vi "Run Test.vi"(8 "error in (no error)":errorcluster, 11 "Test Template in":refnum<class "LCM Single-Up APP Programming.lvclass">) -> (0 "error out":errorcluster, 1 "Fail Codes":string[](array[string]), 2 "Tests Passed":bool[](array[boolean]), 3 "Test Template out":refnum<class "LCM Single-Up APP Programming.lvclass">)   [LabVIEW 2015, in "LCM Single-Up APP Programming.lvclass"]
uses:
  LCM Single-Up APP Programming.lvclass
  Test Class/Test Class.lvclass/Test Class.ctl
  Test Class/Test Class.lvclass
  LCM Single-Up MTS Programming/LCM Single-Up MTS Programming.lvclass
  Classes/Application/Class/Application.lvclass
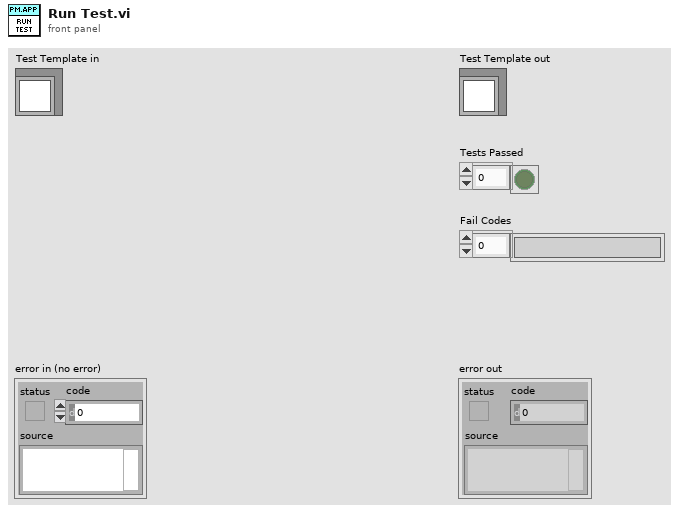
[diagram p1: front panel]
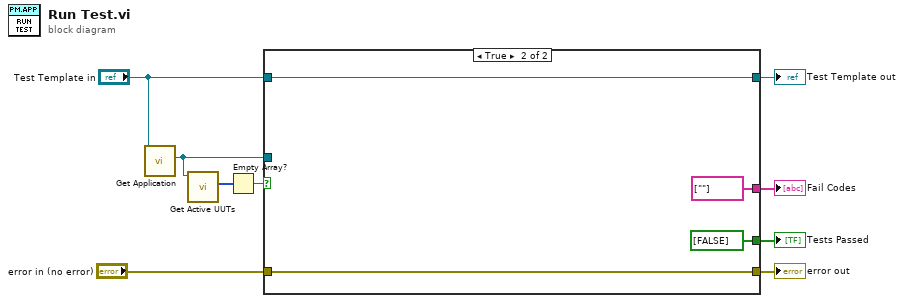
[diagram p0: block diagram]
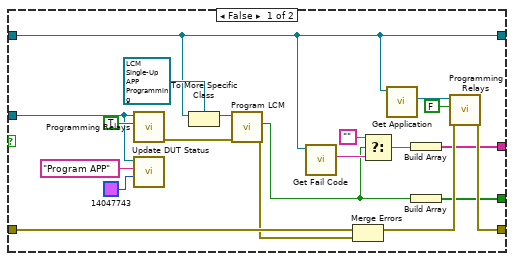
[diagram p2: hidden frame]
diagram:
  n1 = call "Get Application.vi"("Test Class in"="Test Template in") -> ("Application.lvlib:Application.lvclass"=w4:refnum<class "Application.lvclass">)  [unwired: 9 in, 1 out]
  n2 = call "Get Active UUTs.vi"("Application in"=w4) -> ("Active Positions"=w2:u32[])  [unwired: 8 in, 2 out]
  n3 = Empty Array?(array=w2) -> (empty?=w1:bool)
  n4 = case shown="True" w1 {
    tunnel: "error in (no error)" -> [w20 w32]
    tunnel: [w19 w32] -> w8
    tunnel: [w18 string[] [""]] -> w7
    tunnel: [w17 bool[] [FALSE]] -> w6
    tunnel: "Test Template in" -> [w10 w33]
    tunnel: w4 -> [w11 _]
    tunnel: [w10 w33] -> w3
    frame False {
      n5 = call "Programming Relays.vi"("Connect (False)"=TRUE, "Application in"=w11) -> ("error out"=w14:errorcluster)  [unwired: 9 in]
      n6 = call "Update DUT Status.vi"("BG Color"=u32 14047743, "Message ('')"="Program APP", "Application in"=w11) -> ()  [unwired: 7 in, 2 out]
      n7 = To More Specific Class(target class=refnum<class "LCM Single-Up APP Programming.lvclass"> refnum ("LCM Single-Up APP Programming.lvclass"), reference=w10) -> (specific class reference=w15:refnum<class "LCM Single-Up APP Programming.lvclass">)  [unwired: 1 in, 1 out]
      n8 = call "Program LCM.vi"("error in (no error)"=w14, "LCM Single-Up APP Programming in"=w15) -> ("error out"=w12:errorcluster, "Success"=w13:bool)  [unwired: 7 in, 1 out]
      n9 = call "Get Fail Code.vi"("Test Class in"=w10) -> ("Fail Code"=w27:string)  [unwired: 9 in, 1 out]
      n10 = Merge Errors(w20, w12) -> (w21:errorcluster)
      n11 = Select(t="", s=w13, f=w27) -> (s? t:f=w25:string)
      n12 = call "Get Application.vi"("Test Class in"=w10) -> ("Application.lvlib:Application.lvclass"=w28:refnum<class "Application.lvclass">)  [unwired: 9 in, 1 out]
      n13 = Build Array(w25) -> (w18:string[])
      n14 = Build Array(w13) -> (w17:bool[])
      n15 = call "Programming Relays.vi"("error in (no error)"=w21, "Connect (False)"=FALSE, "Application in"=w28) -> ("error out"=w19:errorcluster)  [unwired: 8 in]
    }
    frame True {
    }
  }
  "error out" <- w8
  "Test Template out" <- w3
  "Tests Passed" <- w6
  "Fail Codes" <- w7
